vi "Actor Core.vi"(8 "error in":errorcluster, 11 "Diplom Controller in":refnum<class "Diplom Controller.lvclass">) -> (0 "error out":errorcluster, 3 "Actor out":refnum<class "Actor.lvclass">)   [LabVIEW 2019, in "Diplom Controller.lvlib" / "Diplom Controller.lvclass"]
doc: "(<B>Filename</B>: Actor Framework.lvlib:Actor.lvclass:Actor Core.vi)\n\nReceives messages to the actor, reacts to them, and initiates any error handling that may shut the actor down.\n\nDescendant classes may override this VI to append parallel tasks for the actor to complete while it handles messages. Overrides use the Call Parent Method node."
uses:
  Diplom Controller.lvclass
  C:/Program Files (x86)/National Instruments/LabVIEW 2019/vi.lib/ActorFramework/Actor/Actor.lvclass
  <vilib>/ActorFramework/Actor/Actor.lvclass
  UI Controller/UI Controller/UI Controller.lvclass
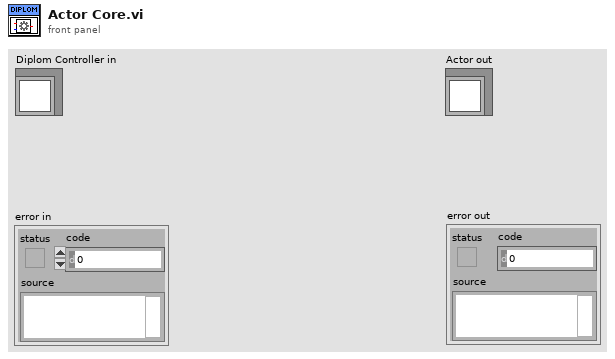
[diagram p1: front panel]
types:
  T1 = enum32{"Invalid", "Standard", "Closed", "Hidden", "Minimized", "Maximized"}
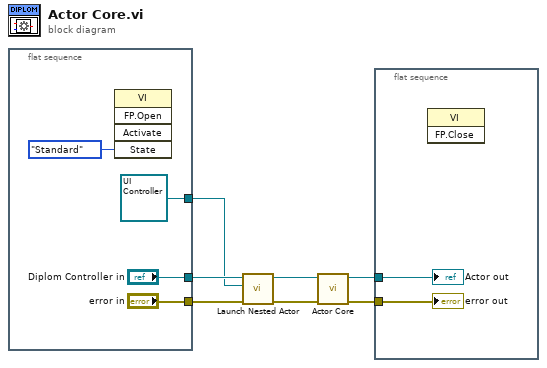
[diagram p0: block diagram]
diagram:
  n1 = flat-sequence {
    tunnel: ["Diplom Controller in"] -> w5
    tunnel: [refnum<class "UI Controller.lvclass"> refnum ("UI Controller.lvlib:UI Controller.lvclass")] -> w4
    tunnel: ["error in"] -> w2
    frame #0 {
      n2 = invoke class="VI" method="FP.Open"("State"=T1."Standard") -> ()  [unwired: 4 in, 5 out]
    }
  }
  n3 = call <vilib>:"Launch Nested Actor.vi"("error in (no error)"=w2, "Nested Actor"=w4, "Caller Actor in"=w5) -> ("error out"=w6:errorcluster, "Caller Actor out"=w3:refnum<class "Diplom Controller.lvclass">)  [unwired: 6 in, 1 out]
  n4 = call-parent "Actor Core.vi"("error in"=w6, "Actor in"=w3) -> ("error out"=w1:errorcluster, "Actor out"=w7:refnum<class "Actor.lvclass">)  [unwired: 8 in]
  n5 = flat-sequence {
    tunnel: w7 -> [w13]
    tunnel: w1 -> [w12]
    frame #0 {
      n6 = invoke class="VI" method="FP.Close"() -> ()  [unwired: 3 in, 3 out]
      "error out" <- w12
      "Actor out" <- w13
    }
  }
